vi "InitCSMs.vi"(7 "Enable Conditional Building lvlibp?":bool=TRUE, 8 "error in":errorcluster, 11 "TestCSMSuite in":refnum<class "TestCSMSuite.lvclass">) -> (0 "error out":errorcluster, 3 "TestCSMSuite out":refnum<class "TestCSMSuite.lvclass">)   [LabVIEW 2017, in "TestCSMSuite.lvclass"]
uses:
  TestCSMSuite.lvclass
  TestCSMSuite.lvclass/TestCSMSuite.ctl
  CSM/Chain1.vi
  CSM/Chain2.vi
  CSM/Chain3.vi
  <vilib>/AppBuilder/AB_API_Simple/Build (path).vi
  CSM/CSM-Testcase.lvlib
  src/user.lib/_NEVSTOP/Communicable State Machine(CSM)/Communicable State Machine.lvlib
  <vilib>/AppBuilder/AB_API_Simple/NI_App_Builder_API.lvlib
panel:
  out "Waited (ms)":u32
  out "CSMs Left":string[](array[string])
  out "Generated files":path[](array[path])
  out "CSMs":string[](array[string])
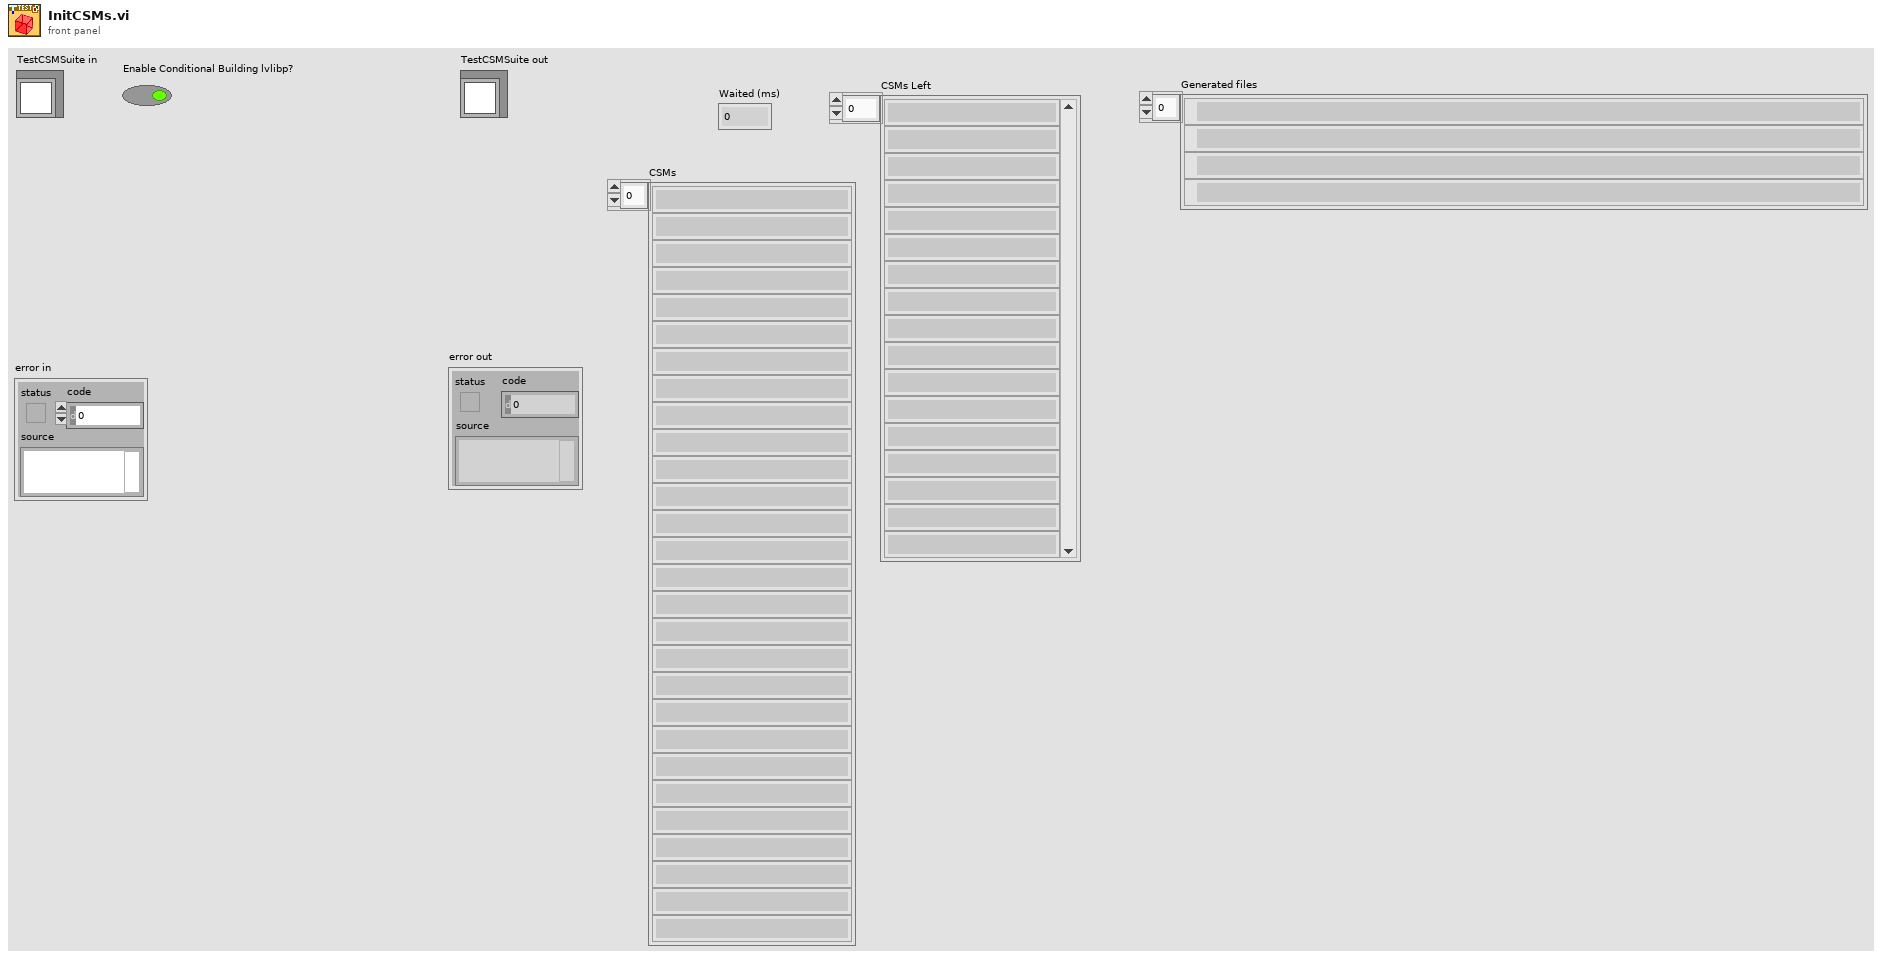
[diagram p1: front panel]
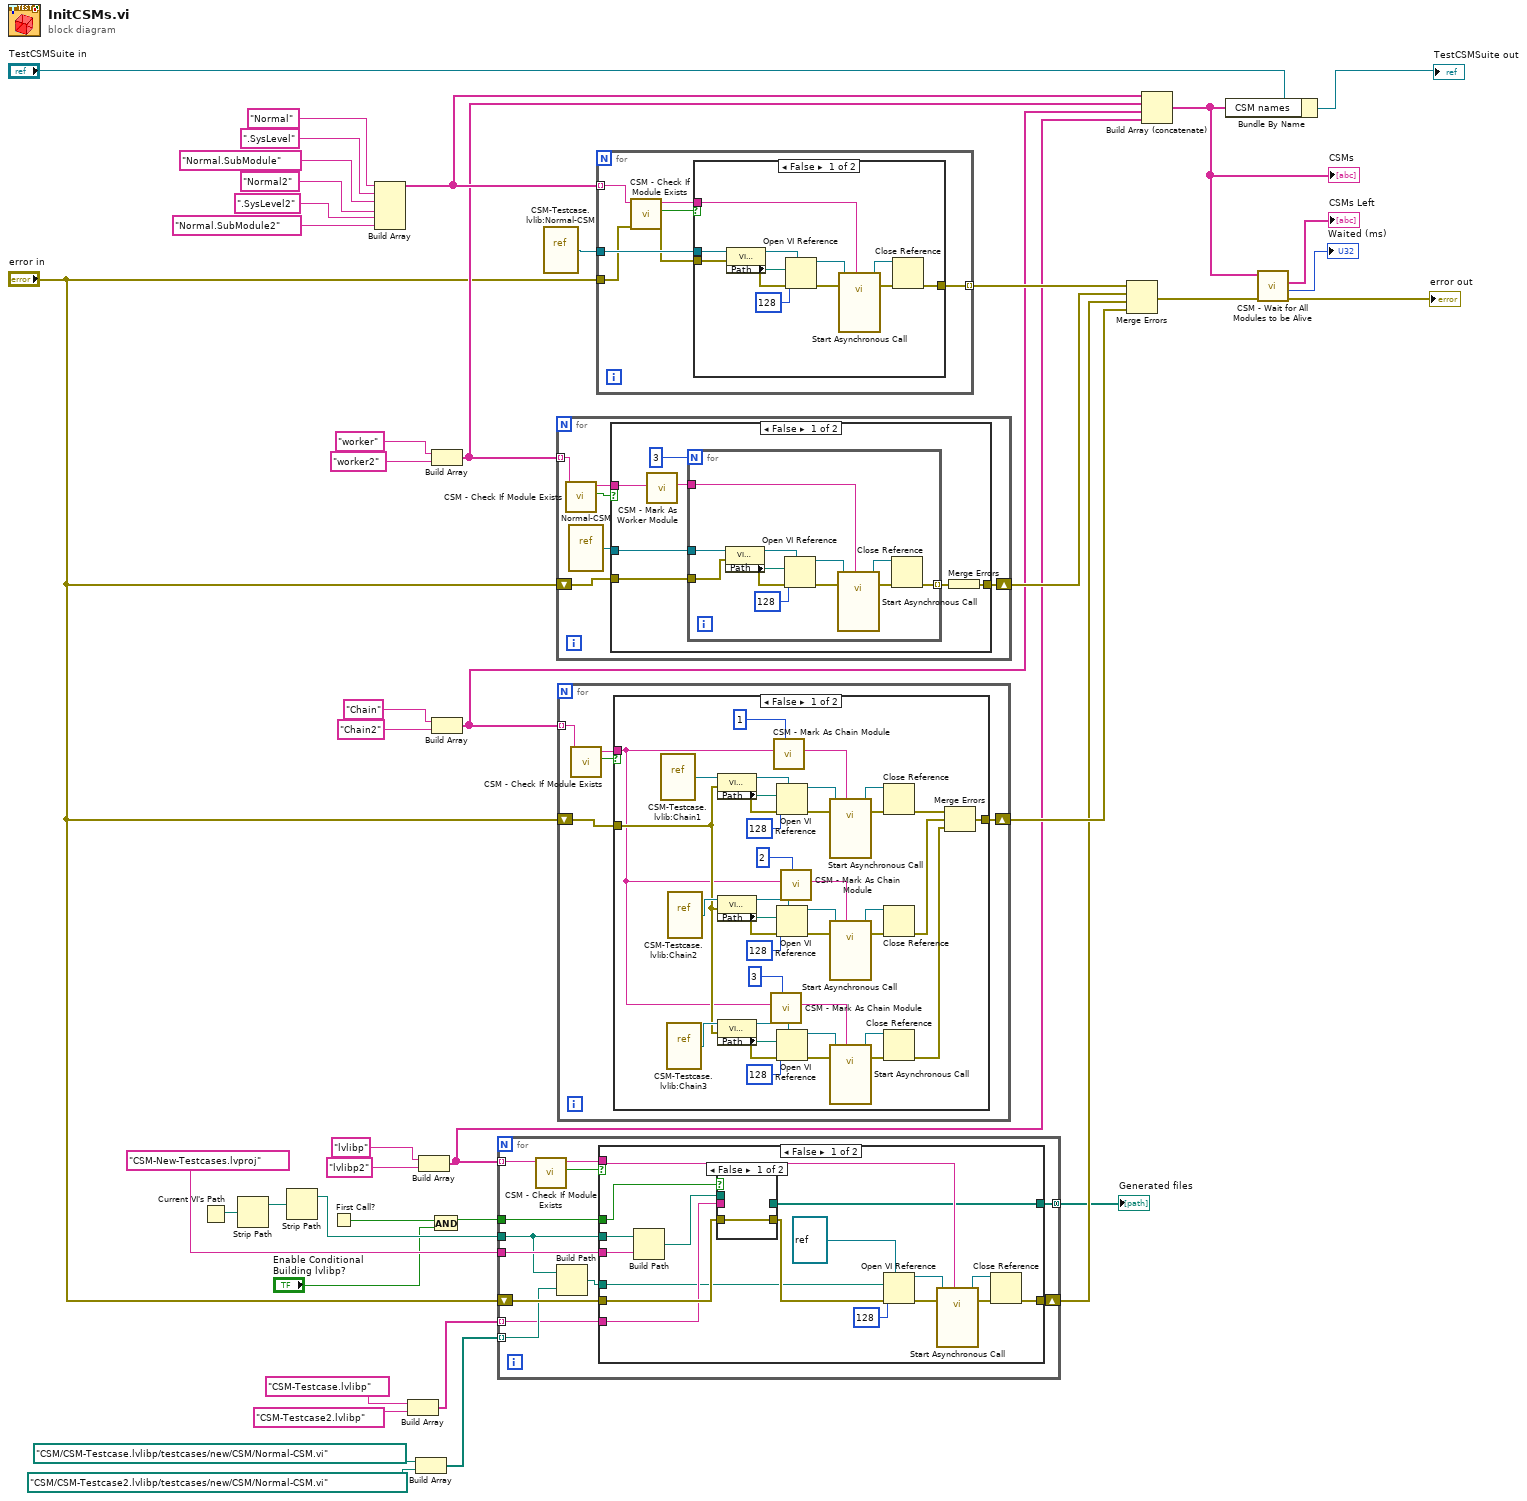
[diagram p0: block diagram]
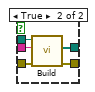
[diagram p2: hidden frame]
diagram:
  n1 = Current VI's Path() -> (path=w39:path)
  n2 = Strip Path(path=w39) -> (stripped path=w40:path)  [unwired: 1 out]
  n3 = Strip Path(path=w40) -> (stripped path=w41:path)  [unwired: 1 out]
  n4 = First Call?() -> (First Call?: T/F=w3:bool)
  n5 = Build Array("Normal" ("Name (\"\" to Use UUID)"), ".SysLevel" ("Name (\"\" to Use UUID)"), "Normal.SubModule" ("Name (\"\" to Use UUID)"), "Normal2" ("Name (\"\" to Use UUID)"), ".SysLevel2" ("Name (\"\" to Use UUID)"), "Normal.SubModule2" ("Name (\"\" to Use UUID)")) -> (w35:string[])
  n6 = Build Array("CSM-Testcase.lvlibp" ("Name of build specification (if empty: build all)"), "CSM-Testcase2.lvlibp" ("Name of build specification (if empty: build all)")) -> (w13:string[])
  n7 = Build Array(path "CSM/CSM-Testcase.lvlibp/testcases/new/CSM/Normal-CSM.vi" ("vi path"), path "CSM/CSM-Testcase2.lvlibp/testcases/new/CSM/Normal-CSM.vi" ("vi path")) -> (w16:path[])
  n8 = Build Array("lvlibp" ("Name (\"\" to Use UUID)"), "lvlibp2" ("Name (\"\" to Use UUID)")) -> (w19:string[])
  n9 = And(x=w3, y="Enable Conditional Building lvlibp?") -> (x .and. y?=w2:bool)
  n10 = Build Array("worker" ("Name (\"\" to Use UUID)"), "worker2" ("Name (\"\" to Use UUID)")) -> (w25:string[])
  n11 = Build Array("Chain" ("Name (\"\" to Use UUID)"), "Chain2" ("Name (\"\" to Use UUID)")) -> (w22:string[])
  n12 = for {
    tunnel: "CSM-New-Testcases.lvproj" ("name or relative path") -> [w53]
    tunnel: w41 -> [w48]
    shift-right: [w52] -> w38
    shift-left: "error in" -> [w54]
    tunnel: w19 -> [w50] mode=indexing
    tunnel: w16 -> [w49] mode=indexing
    tunnel: w13 -> [w46] mode=indexing
    tunnel: [w45] -> w12 mode=concatenating
    tunnel: w2 -> [w44]
    n13 = call "CSM - Check If Module Exists.vi"("CSM Name"=w50) -> ("Exist?"=w55:bool, "CSM Name (Dup)"=w51:string)  [unwired: 8 in, 1 out]
    n14 = Build Path(base path=w48, name or relative path=w49) -> (appended path=w47:path)
    n15 = case shown="False" w55 {
      tunnel: [w72 w79] -> w52
      tunnel: w47 -> [w58 _]
      tunnel: w48 -> [w65 _]
      tunnel: w53 -> [w64 _]
      tunnel: w51 -> [w63 _]
      tunnel: w54 -> [w62 w79]
      tunnel: w46 -> [w60 _]
      tunnel: [w59 _] -> w45
      tunnel: w44 -> [w56 _]
      frame False {
        n16 = Build Path(base path=w65, name or relative path=w64) -> (appended path=w57:path)
        n17 = case shown="False" w56 {
          tunnel: w62 -> [w73 w78]
          tunnel: [w73 w77] -> w61
          tunnel: w60 -> [_ w76]
          tunnel: [_ w75] -> w59
          tunnel: w57 -> [_ w74]
          frame False {
          }
          frame True {
            n18 = call-poly <vilib>:"Build.vi"("error in (no error)"=w78, "Name of build specification (if empty: build all)"=w76, "Path to project"=w74) -> ("error out"=w77:errorcluster, "Generated files"=w75:path[])  [unwired: 7 in]
          }
        }
        n19 = Open VI Reference(type specifier VI Refnum (for type only)=refnum<vi> refnum ("reference out"), vi path=w58, options=128, error in (no error)=w61) -> (vi reference=w68:refnum<vi>, error out=w70:errorcluster)  [unwired: 2 in]
        n20 = call-by-ref "Start Asynchronous Call"(reference=w68, error in=w70, "Name (\"\" to Use UUID)"=w63) -> (reference out=w67:refnum<vi>, error out=w69:errorcluster)  [unwired: 11 in]
        n21 = Close Reference(reference=w67, error in (no error)=w69) -> (error out=w72:errorcluster)
      }
      frame True {
      }
    }
  }
  "Generated files" <- w12
  n22 = vi-ref "CSM-Testcase.lvlib:Normal-CSM.vi"() -> (w31:refnum<vi>)
  n23 = for {
    shift-right: [w82] -> w37
    shift-left: "error in" -> [w85]
    tunnel: w25 -> [w81] mode=indexing
    n24 = call "CSM - Check If Module Exists.vi"("CSM Name"=w81) -> ("Exist?"=w84:bool, "CSM Name (Dup)"=w83:string)  [unwired: 8 in, 1 out]
    n25 = vi-ref "Normal-CSM.vi"() -> (w80:refnum<vi>)
    n26 = case shown="False" w84 {
      tunnel: w80 -> [w92 _]
      tunnel: [w86 w105] -> w82
      tunnel: w85 -> [w88 w105]
      tunnel: w83 -> [w87 _]
      frame False {
        n27 = call "CSM - Mark As Worker Module.vi"("CSM Name"=w87) -> ("CSM Name (Marked As Worker)"=w89:string)  [unwired: 9 in]
        n28 = for {
          N: 3 -> [_]
          tunnel: w92 -> [w96]
          tunnel: w89 -> [w95]
          tunnel: [w94] -> w90 mode=indexing
          tunnel: w88 -> [w93]
          n29 = property class="VI (strict)"(reference=w96, error in=w93) -> (reference out=w102:refnum<vi>, error out=w100:errorcluster, "Path"=w99:path)
          n30 = Open VI Reference(type specifier VI Refnum (for type only)=w102, vi path=w99, options=128, error in (no error)=w100) -> (vi reference=w98:refnum<vi>, error out=w103:errorcluster)  [unwired: 2 in]
          n31 = call-by-ref "Start Asynchronous Call"(reference=w98, error in=w103, "Name (\"\" to Use UUID)"=w95) -> (reference out=w97:refnum<vi>, error out=w101:errorcluster)  [unwired: 11 in]
          n32 = Close Reference(reference=w97, error in (no error)=w101) -> (error out=w94:errorcluster)
        }
        n33 = Merge Errors(w90) -> (w86:errorcluster)
      }
      frame True {
      }
    }
  }
  n34 = for {
    shift-right: [w108] -> w43
    shift-left: "error in" -> [w110]
    tunnel: w22 -> [w106] mode=indexing
    n35 = call "CSM - Check If Module Exists.vi"("CSM Name"=w106) -> ("Exist?"=w109:bool, "CSM Name (Dup)"=w107:string)  [unwired: 8 in, 1 out]
    n36 = case shown="False" w109 {
      tunnel: [w113 w150] -> w108
      tunnel: w110 -> [w112 w150]
      tunnel: w107 -> [w111 _]
      frame False {
        n37 = vi-ref "CSM-Testcase.lvlib:Chain1.vi"() -> (w149:refnum<vi>)
        n38 = vi-ref "CSM-Testcase.lvlib:Chain3.vi"() -> (w131:refnum<vi>)
        n39 = vi-ref "CSM-Testcase.lvlib:Chain2.vi"() -> (w132:refnum<vi>)
        n40 = property class="VI (strict)"(reference=w149, error in=w112) -> (reference out=w146:refnum<vi>, error out=w144:errorcluster, "Path"=w143:path)
        n41 = property class="VI (strict)"(reference=w132, error in=w112) -> (reference out=w135:refnum<vi>, error out=w137:errorcluster, "Path"=w138:path)
        n42 = property class="VI (strict)"(reference=w131, error in=w112) -> (reference out=w128:refnum<vi>, error out=w126:errorcluster, "Path"=w125:path)
        n43 = call "CSM - Mark As Chain Module.vi"("Order"=3, "CSM Name"=w111) -> ("CSM Name (Marked As Chain)"=w119:string)  [unwired: 8 in]
        n44 = call "CSM - Mark As Chain Module.vi"("Order"=1, "CSM Name"=w111) -> ("CSM Name (Marked As Chain)"=w117:string)  [unwired: 8 in]
        n45 = Open VI Reference(type specifier VI Refnum (for type only)=w146, vi path=w143, options=128, error in (no error)=w144) -> (vi reference=w142:refnum<vi>, error out=w147:errorcluster)  [unwired: 2 in]
        n46 = Open VI Reference(type specifier VI Refnum (for type only)=w135, vi path=w138, options=128, error in (no error)=w137) -> (vi reference=w139:refnum<vi>, error out=w134:errorcluster)  [unwired: 2 in]
        n47 = Open VI Reference(type specifier VI Refnum (for type only)=w128, vi path=w125, options=128, error in (no error)=w126) -> (vi reference=w124:refnum<vi>, error out=w129:errorcluster)  [unwired: 2 in]
        n48 = call "CSM - Mark As Chain Module.vi"("Order"=2, "CSM Name"=w111) -> ("CSM Name (Marked As Chain)"=w118:string)  [unwired: 8 in]
        n49 = call-by-ref "Start Asynchronous Call"(reference=w142, error in=w147, "Name (\"\" to Use UUID)"=w117) -> (reference out=w141:refnum<vi>, error out=w145:errorcluster)  [unwired: 11 in]
        n50 = call-by-ref "Start Asynchronous Call"(reference=w139, error in=w134, "Name (\"\" to Use UUID)"=w118) -> (reference out=w140:refnum<vi>, error out=w136:errorcluster)  [unwired: 11 in]
        n51 = call-by-ref "Start Asynchronous Call"(reference=w124, error in=w129, "Name (\"\" to Use UUID)"=w119) -> (reference out=w123:refnum<vi>, error out=w127:errorcluster)  [unwired: 11 in]
        n52 = Close Reference(reference=w141, error in (no error)=w145) -> (error out=w122:errorcluster)
        n53 = Close Reference(reference=w140, error in (no error)=w136) -> (error out=w121:errorcluster)
        n54 = Close Reference(reference=w123, error in (no error)=w127) -> (error out=w120:errorcluster)
        n55 = Merge Errors(w122, w121, w120) -> (w113:errorcluster)
      }
      frame True {
      }
    }
  }
  n56 = for {
    tunnel: w31 -> [w157]
    tunnel: w35 -> [w153] mode=indexing
    tunnel: [w156] -> w36 mode=indexing
    tunnel: "error in" -> [w155]
    n57 = call "CSM - Check If Module Exists.vi"("Error In"=w155, "CSM Name"=w153) -> ("error out"=w154:errorcluster, "Exist?"=w151:bool, "CSM Name (Dup)"=w152:string)  [unwired: 7 in]
    n58 = case shown="False" w151 {
      tunnel: w157 -> [w161 _]
      tunnel: [w160 w170] -> w156
      tunnel: w154 -> [w159 w170]
      tunnel: w152 -> [w158 _]
      frame False {
        n59 = property class="VI (strict)"(reference=w161, error in=w159) -> (reference out=w167:refnum<vi>, error out=w165:errorcluster, "Path"=w164:path)
        n60 = Open VI Reference(type specifier VI Refnum (for type only)=w167, vi path=w164, options=128, error in (no error)=w165) -> (vi reference=w163:refnum<vi>, error out=w168:errorcluster)  [unwired: 2 in]
        n61 = call-by-ref "Start Asynchronous Call"(reference=w163, error in=w168, "Name (\"\" to Use UUID)"=w158) -> (reference out=w162:refnum<vi>, error out=w166:errorcluster)  [unwired: 11 in]
        n62 = Close Reference(reference=w162, error in (no error)=w166) -> (error out=w160:errorcluster)
      }
      frame True {
      }
    }
  }
  n63 = Merge Errors(w36, w37, w38, w43) -> (w11:errorcluster)
  n64 = Build Array (concatenate)(w35, w25, w22, w19) -> (w10:string[])
  "CSMs" <- w10
  n65 = Bundle By Name(cluster="TestCSMSuite in", "CSM names"=w10) -> (→"TestCSMSuite out":refnum<class "TestCSMSuite.lvclass">)
  n66 = call "CSM - Wait for All Modules to be Alive.vi"("Error In"=w11, "CSM Names"=w10) -> ("error out"=→"error out":errorcluster, "Waited (ms)"=→"Waited (ms)":u32, "CSMs Left"=→"CSMs Left":string[])  [unwired: 7 in]
